vi "AnyBuilderBuildToBuffer.vi"(8 "error in":errorcluster, 10 "Message Type":string, 11 "Builder Ref":T1) -> (0 "error out":errorcluster, 3 "Buffer":u8[](array[numeric]))   [LabVIEW 2019, in "grpc-lvsupport.lvlib"]
uses:
  grpc-lvsupport.lvlib
  grpcId.ctl
  <vilib>/Utility/error.llb/Error Cluster From Error Code.vi
  <resource>/labview_grpc_server.dll
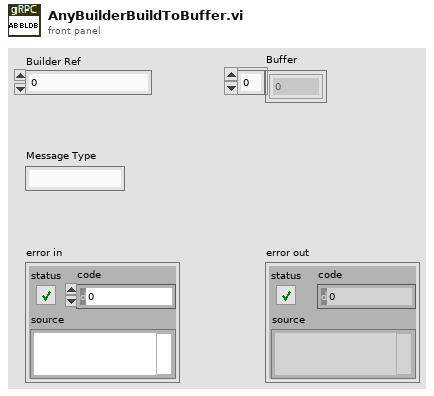
[diagram p1: front panel]
types:
  T1 = typedef "grpc-lvsupport.lvlib/grpcId.ctl" = u64
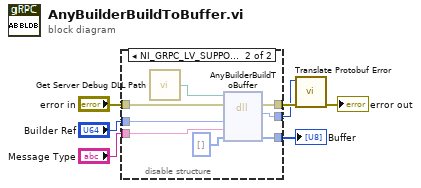
[diagram p0: block diagram]
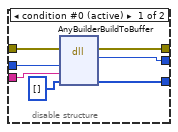
[diagram p2: hidden frame]
diagram:
  n1 = disable-structure shown="NI_GRPC_LV_SUPPORT_DEBUG==True&&RUN_TIME_ENGINE==False" {
    disable-tunnel: "error in" -> [w14 w22]
    disable-tunnel: [w13 w21] -> w6
    disable-tunnel: "Builder Ref" -> [w12 w19]
    disable-tunnel: "Message Type" -> [w11 w18]
    disable-tunnel: [w10 w17] -> w3
    disable-tunnel: [w9 w16] -> w1
    frame condition #0 (active) {
      n2 = dll-call lib="C:/Program Files (x86)/National Instruments/LabVIEW 2024/resource/labview_grpc_server.*" fn="AnyBuilderBuildToBuffer"(error in=w14, "builderId"=w12, "messageType"=w11, "anyId"=u8[] []) -> (error out=w13:errorcluster, "return type"=w9:i32, "anyId"=w10:u8[])  [unwired: 4 in, 1 out]
    }
    frame condition #1 {
      n3 = call "Get Server Debug DLL Path.vi"() -> ("DLL Path"=w20:path)
      n4 = dll-call lib="?" fn="AnyBuilderBuildToBuffer"(path in=w20, error in=w22, "builderId"=w19, "messageType"=w18, "anyId"=u8[] []) -> (error out=w21:errorcluster, "return type"=w16:i32, "anyId"=w17:u8[])  [unwired: 3 in, 1 out]
    }
  }
  "Buffer" <- w3
  n5 = call "Translate Protobuf Error.vi"("error in"=w6, "Error Code"=w1) -> ("error out"=→"error out":errorcluster)  [unwired: 9 in]
